vi "DO driver motor.vi"() -> ()   [LabVIEW 2017]
panel:
  in  "Stop":bool
  in  "Start":bool
  in  "Down":bool
  in  "Up":bool
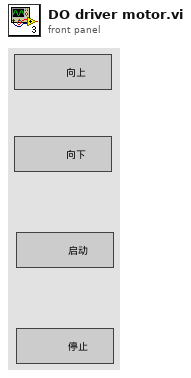
[diagram p1: front panel]
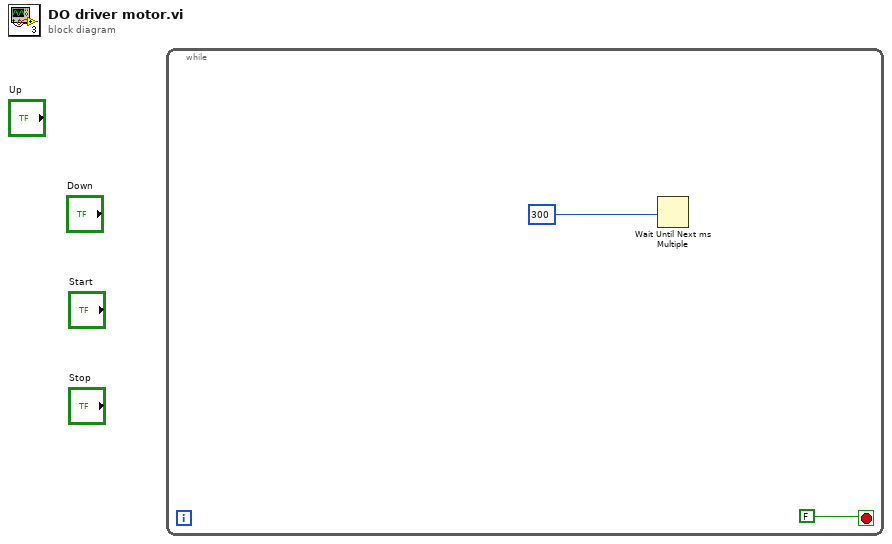
[diagram p0: block diagram]
diagram:
  n1 = while {
    stop <- FALSE stop-if-true
    n2 = Wait Until Next ms Multiple(millisecond multiple=300) -> ()  [unwired: 1 out]
  }
